vi "MarkerSabtract (SubVI).vi"(1 "B":T1, 2 "A":T1) -> (0 "A-B":dbl[](array[numeric]))   [LabVIEW 2021]
uses:
  ctrOWLMarker.ctl
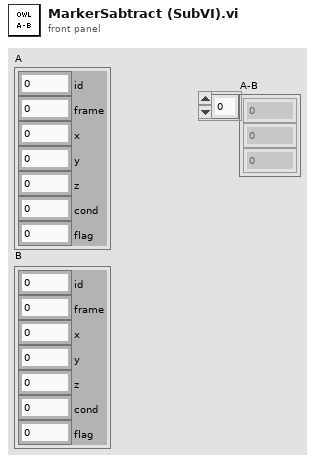
[diagram p1: front panel]
types:
  T1 = typedef "ctrOWLMarker.ctl" = cluster{"id":i32, "frame":i32, "x":sgl, "y":sgl, "z":sgl, "cond":sgl, "flag":u32}
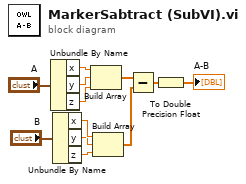
[diagram p0: block diagram]
diagram:
  n1 = Unbundle By Name("A") -> ("x"=w3:sgl, "y"=w4:sgl, "z"=w5:sgl)
  n2 = Unbundle By Name("B") -> ("x"=w9:sgl, "y"=w8:sgl, "z"=w7:sgl)
  n3 = Build Array(w3, w4, w5) -> (w12:sgl[])
  n4 = Build Array(w9, w8, w7) -> (w11:sgl[])
  n5 = Subtract(x=w12, y=w11) -> (x-y=w2:sgl[])
  n6 = To Double Precision Float(number=w2) -> (double precision float=→"A-B":dbl[])
